vi "SO2 TCP Packet_v3.1.vi"(0 "ID":string, 5 "Version":string, 7 "TCP Packet In":string, 9 "utc_time":u32, 13 "Data Array":string[](array[string])) -> (8 "TCP Binary Packet":string)   [LabVIEW 2014]
panel:
  out "array":string[](array[string])
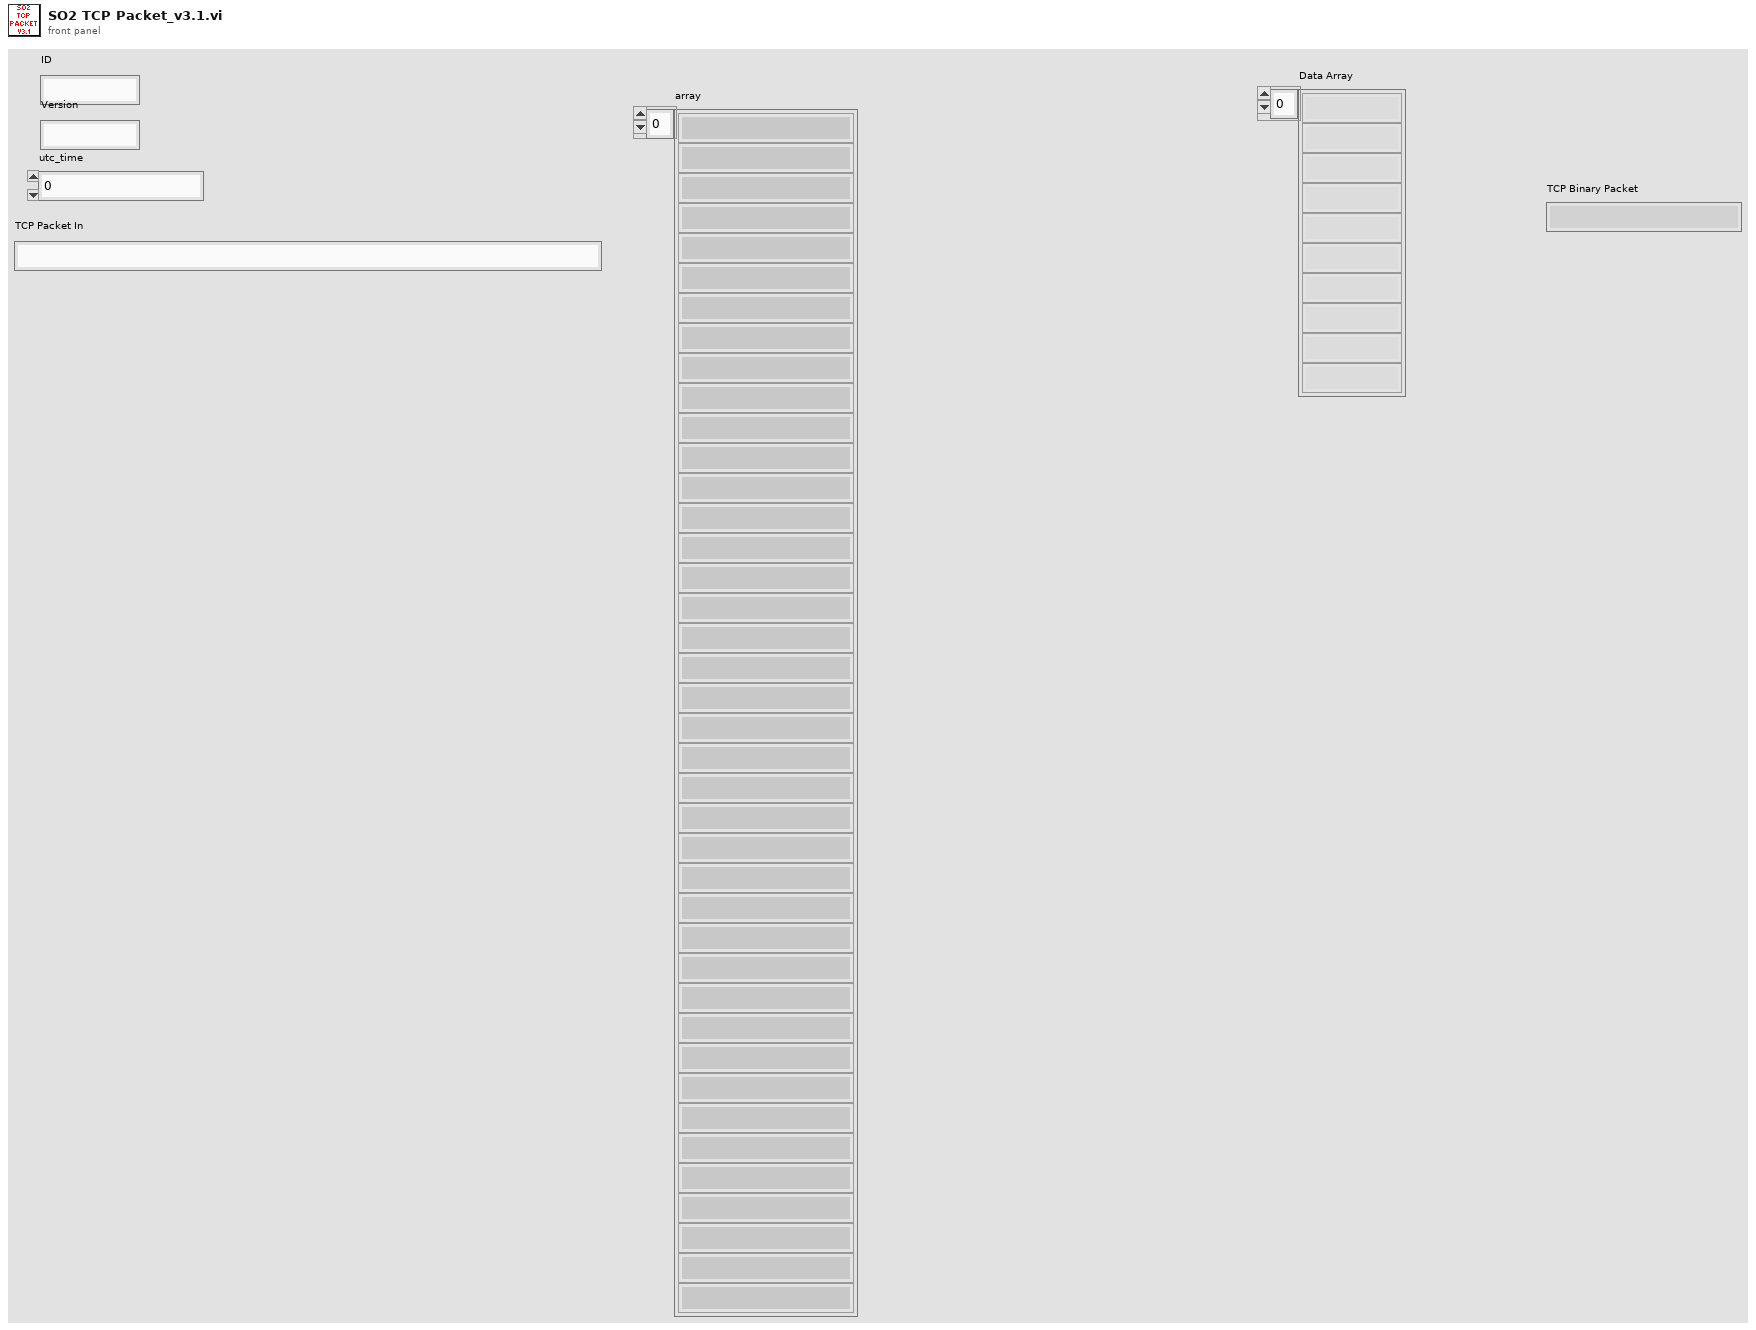
[diagram p1: front panel]
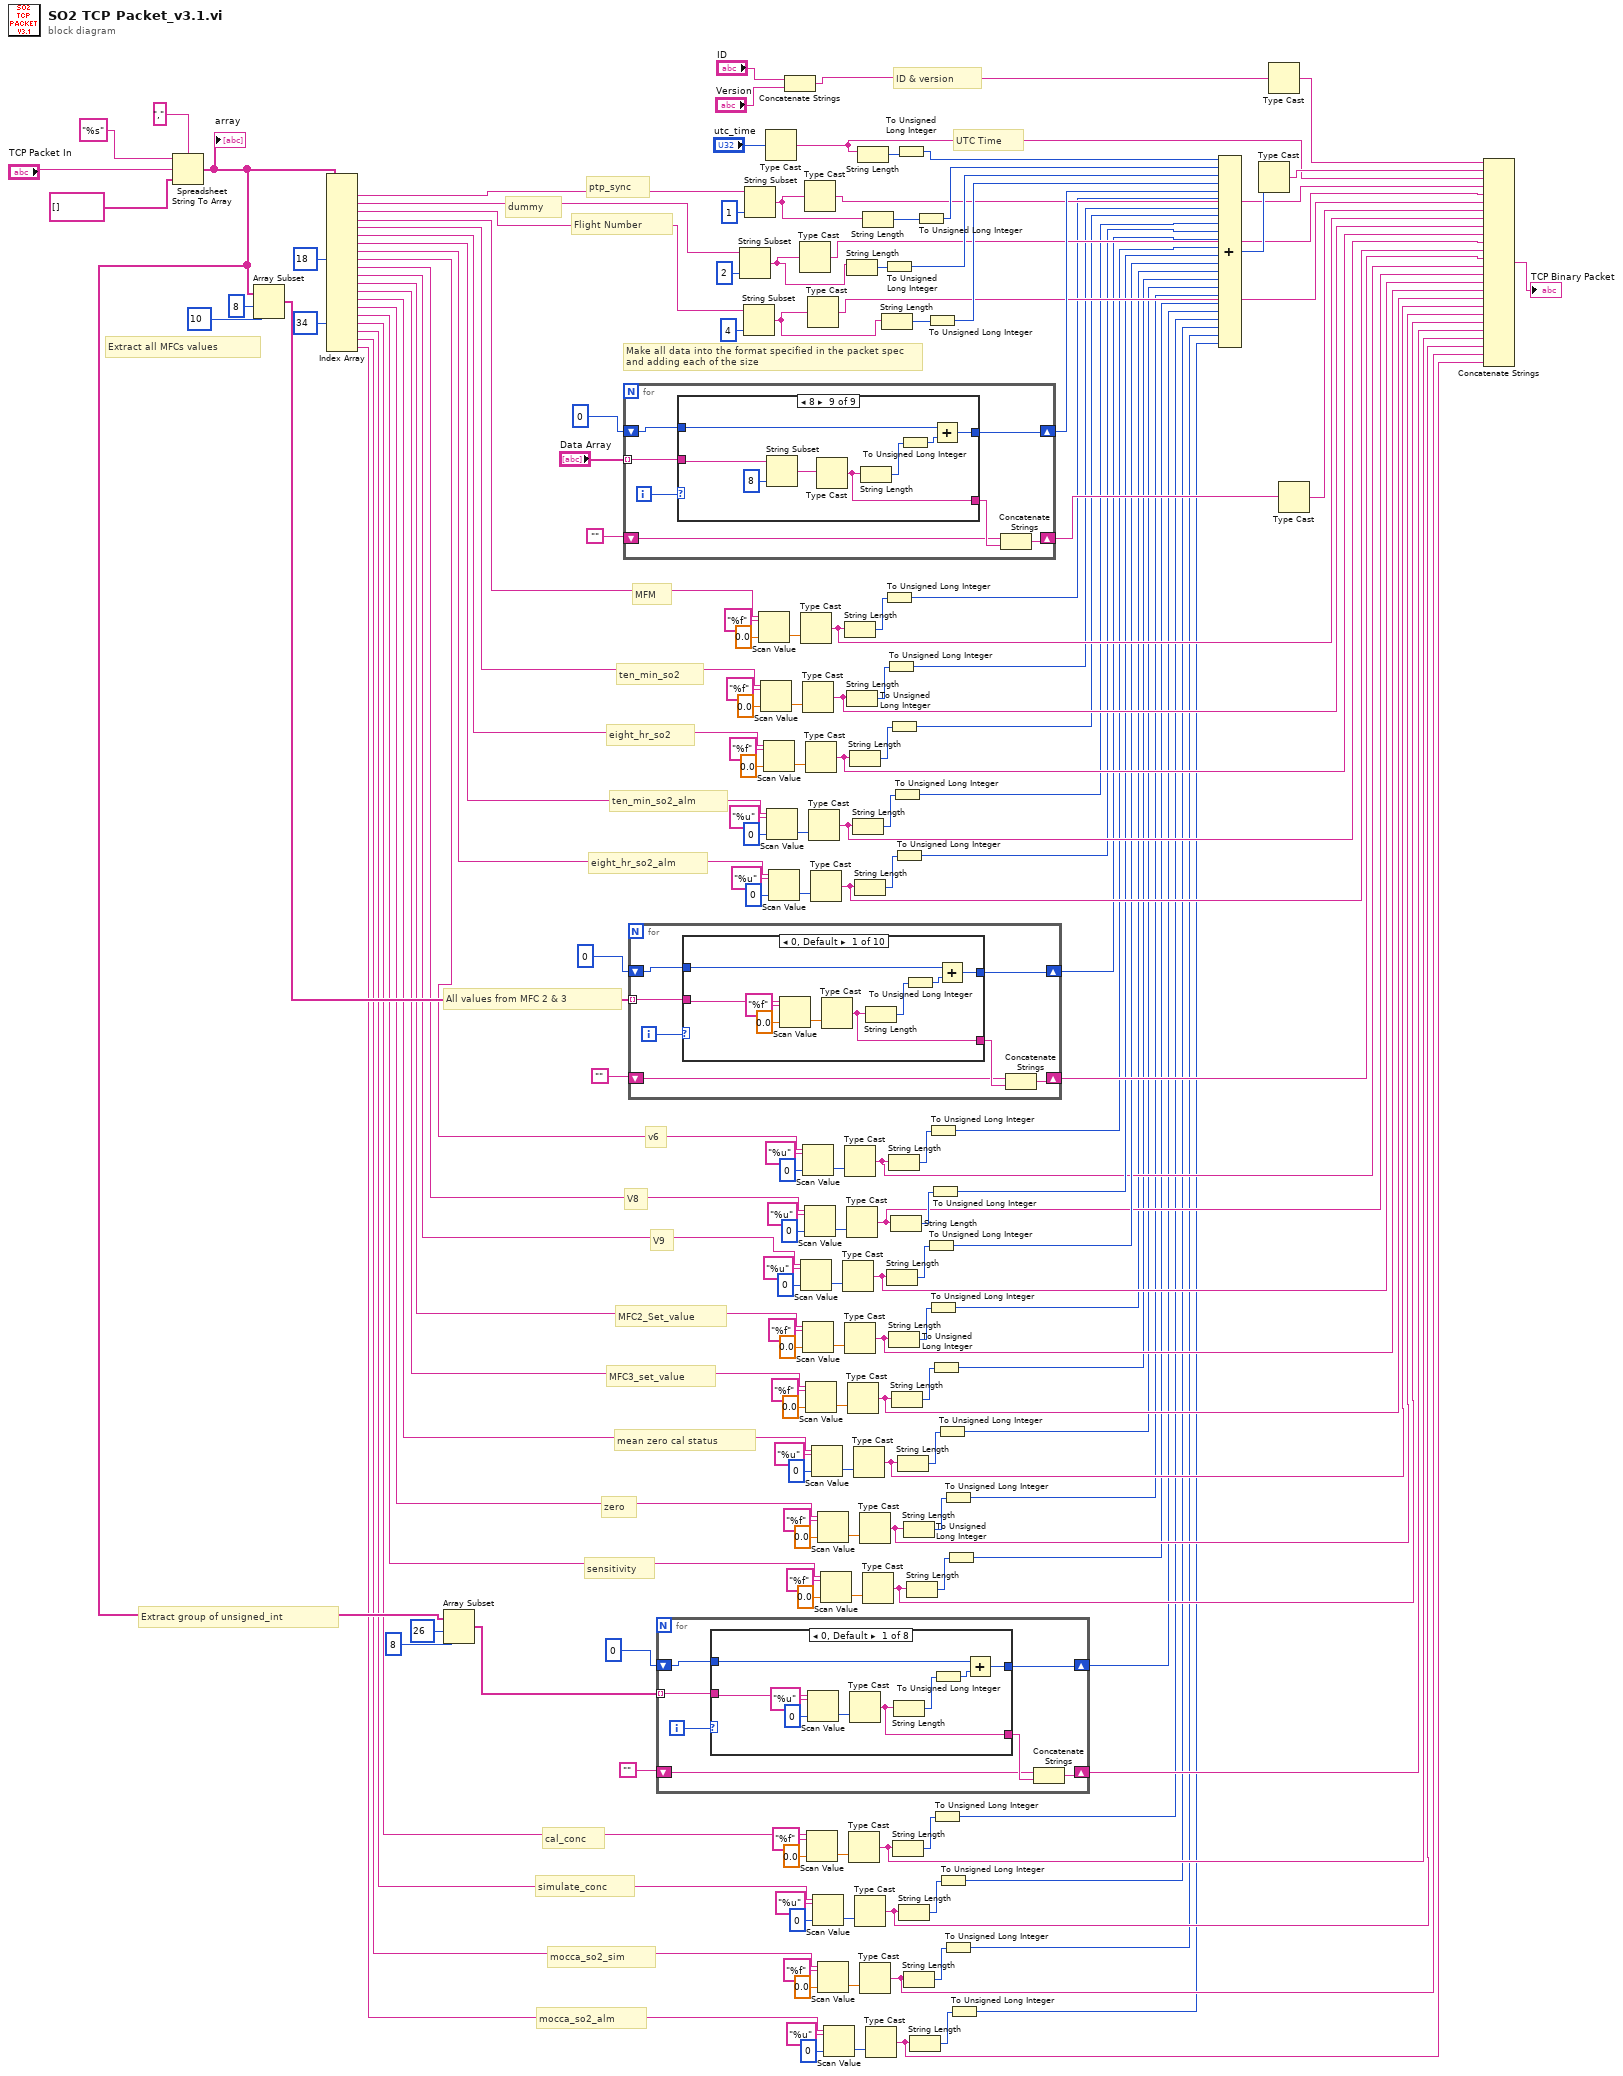
[diagram p0: block diagram]
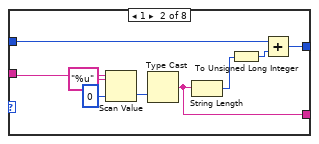
[diagram p2: hidden frame]
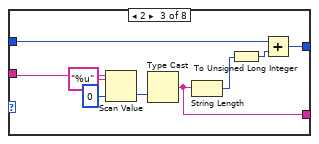
[diagram p3: hidden frame]
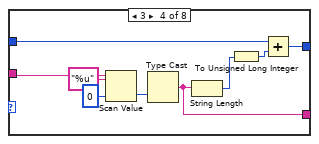
[diagram p4: hidden frame]
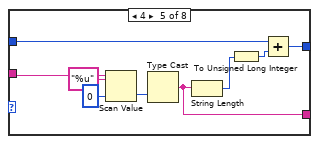
[diagram p5: hidden frame]
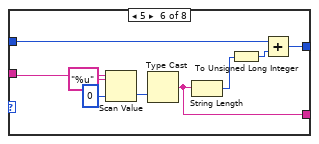
[diagram p6: hidden frame]
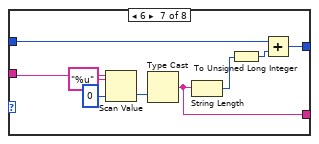
[diagram p7: hidden frame]
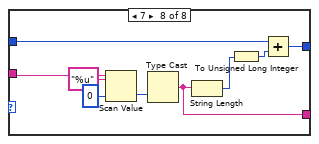
[diagram p8: hidden frame]
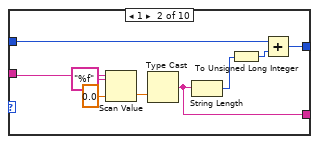
[diagram p9: hidden frame]
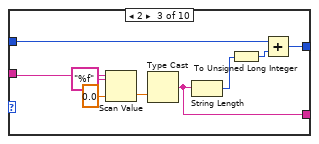
[diagram p10: hidden frame]
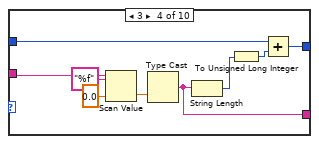
[diagram p11: hidden frame]
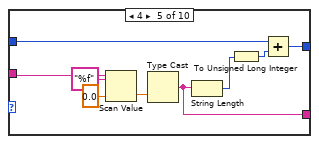
[diagram p12: hidden frame]
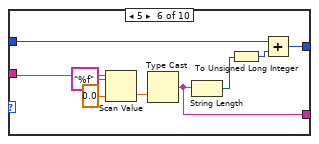
[diagram p13: hidden frame]
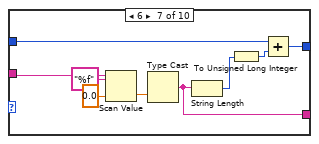
[diagram p14: hidden frame]
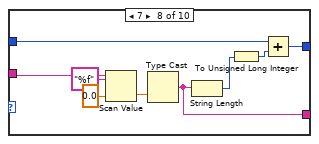
[diagram p15: hidden frame]
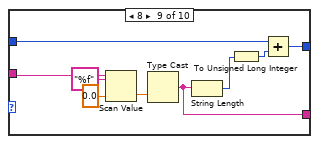
[diagram p16: hidden frame]
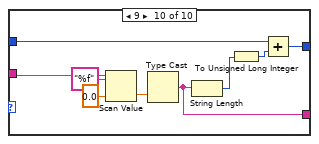
[diagram p17: hidden frame]
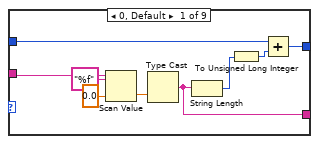
[diagram p18: hidden frame]
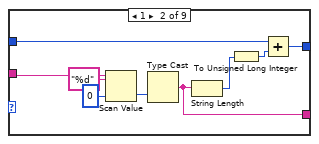
[diagram p19: hidden frame]
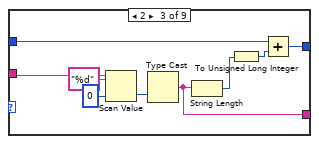
[diagram p20: hidden frame]
diagram:
  # "mocca_so2_alm"
  # "mocca_so2_sim"
  # "simulate_conc"
  # "cal_conc"
  # "Extract group of unsigned_int"
  # "sensitivity"
  # "zero"
  # "mean zero cal status"
  # "MFC3_set_value"
  # "MFC2_Set_value"
  # "V9"
  # "V8"
  # "v6"
  # "All values from MFC 2 & 3"
  # "Extract all MFCs values"
  # "eight_hr_so2_alm"
  # "ten_min_so2_alm"
  # "eight_hr_so2"
  # "ten_min_so2"
  # "MFM"
  # "Flight Number"
  # "dummy"
  # "ptp_sync"
  # "UTC Time"
  # "ID & version"
  # "Make all data into the format specified in the packet spec\nand adding each of the size"
  n1 = Spreadsheet String To Array(delimiter (Tab)=",", format string="%s", spreadsheet string="TCP Packet In", array type (2D Dbl)=string[] []) -> (array=w40:string[])
  "array" <- w40
  n2 = Array Subset(array=w40, index=8, length=10) -> (w102:string[])
  n3 = Index Array(array=w40, index #9=18 ("index"), index #17=34 ("index")) -> (element #1=w144:string, element #2=w143:string, element #3=w142:string, element #4=w137:string, element #5=w126:string, element #6=w123:string, element #7=w112:string, element #8=w109:string, element #9=w90:string, element #10=w89:string, element #11=w84:string, element #12=w69:string, element #13=w64:string, element #14=w59:string, element #15=w48:string, element #16=w43:string, element #17=w17:string, element #18=w8:string, element #19=w7:string, element #20=w6:string)  [unwired: 18 in]
  n4 = Array Subset(array=w40, index=26, length=8) -> (w36:string[])
  n5 = for {
    tunnel: "Data Array" -> [w181] mode=indexing
    shift-right: [w179] -> w163
    shift-left: u32 0 -> [w180]
    shift-right: [w178] -> w152
    shift-left: "" -> [w176]
    i -> [w182]
    n6 = case shown="8" w182 {
      tunnel: w181 -> [w189 w198 w207 w216 w225 w234 w243 w252 w256]
      tunnel: w180 -> [w187 w196 w205 w214 w223 w232 w241 w250 w262]
      tunnel: [w184 w193 w202 w211 w220 w229 w238 w247 w259] -> w179
      tunnel: [w183 w192 w201 w210 w219 w228 w237 w246 w258] -> w177
      frame 0, Default {
        n7 = Scan Value(string=w189, format string="%f", default (0 dbl)=sgl 0.0 ("default (0 I32)")) -> (value=w191:sgl)  [unwired: 1 out]
        n8 = Type Cast(x=w191) -> (*(type *) &x=w183:string)  [unwired: 1 in]
        n9 = String Length(string=w183) -> (length=w186:i32)
        n10 = To Unsigned Long Integer(number=w186) -> (unsigned 32bit integer=w185:u32)
        n11 = Add(x=w187, y=w185) -> (x+y=w184:u32)
      }
      frame 1 {
        n12 = Scan Value(string=w198, format string="%d", default (0 dbl)=0 ("default (0 I32)")) -> (value=w200:i32)  [unwired: 1 out]
        n13 = Type Cast(x=w200) -> (*(type *) &x=w192:string)  [unwired: 1 in]
        n14 = String Length(string=w192) -> (length=w195:i32)
        n15 = To Unsigned Long Integer(number=w195) -> (unsigned 32bit integer=w194:u32)
        n16 = Add(x=w196, y=w194) -> (x+y=w193:u32)
      }
      frame 2 {
        n17 = Scan Value(string=w207, format string="%d", default (0 dbl)=0 ("default (0 I32)")) -> (value=w209:i32)  [unwired: 1 out]
        n18 = Type Cast(x=w209) -> (*(type *) &x=w201:string)  [unwired: 1 in]
        n19 = String Length(string=w201) -> (length=w204:i32)
        n20 = To Unsigned Long Integer(number=w204) -> (unsigned 32bit integer=w203:u32)
        n21 = Add(x=w205, y=w203) -> (x+y=w202:u32)
      }
      frame 3 {
        n22 = Scan Value(string=w216, format string="%d", default (0 dbl)=0 ("default (0 I32)")) -> (value=w218:i32)  [unwired: 1 out]
        n23 = Type Cast(x=w218) -> (*(type *) &x=w210:string)  [unwired: 1 in]
        n24 = String Length(string=w210) -> (length=w213:i32)
        n25 = To Unsigned Long Integer(number=w213) -> (unsigned 32bit integer=w212:u32)
        n26 = Add(x=w214, y=w212) -> (x+y=w211:u32)
      }
      frame 4 {
        n27 = Scan Value(string=w225, format string="%f", default (0 dbl)=sgl 0.0 ("default (0 I32)")) -> (value=w227:sgl)  [unwired: 1 out]
        n28 = Type Cast(x=w227) -> (*(type *) &x=w219:string)  [unwired: 1 in]
        n29 = String Length(string=w219) -> (length=w222:i32)
        n30 = To Unsigned Long Integer(number=w222) -> (unsigned 32bit integer=w221:u32)
        n31 = Add(x=w223, y=w221) -> (x+y=w220:u32)
      }
      frame 5 {
        n32 = Scan Value(string=w234, format string="%f", default (0 dbl)=sgl 0.0 ("default (0 I32)")) -> (value=w236:sgl)  [unwired: 1 out]
        n33 = Type Cast(x=w236) -> (*(type *) &x=w228:string)  [unwired: 1 in]
        n34 = String Length(string=w228) -> (length=w231:i32)
        n35 = To Unsigned Long Integer(number=w231) -> (unsigned 32bit integer=w230:u32)
        n36 = Add(x=w232, y=w230) -> (x+y=w229:u32)
      }
      frame 6 {
        n37 = Scan Value(string=w243, format string="%f", default (0 dbl)=sgl 0.0 ("default (0 I32)")) -> (value=w245:sgl)  [unwired: 1 out]
        n38 = Type Cast(x=w245) -> (*(type *) &x=w237:string)  [unwired: 1 in]
        n39 = String Length(string=w237) -> (length=w240:i32)
        n40 = To Unsigned Long Integer(number=w240) -> (unsigned 32bit integer=w239:u32)
        n41 = Add(x=w241, y=w239) -> (x+y=w238:u32)
      }
      frame 7 {
        n42 = Scan Value(string=w252, format string="%f", default (0 dbl)=sgl 0.0 ("default (0 I32)")) -> (value=w254:sgl)  [unwired: 1 out]
        n43 = Type Cast(x=w254) -> (*(type *) &x=w246:string)  [unwired: 1 in]
        n44 = String Length(string=w246) -> (length=w249:i32)
        n45 = To Unsigned Long Integer(number=w249) -> (unsigned 32bit integer=w248:u32)
        n46 = Add(x=w250, y=w248) -> (x+y=w247:u32)
      }
      frame 8 {
        n47 = String Subset(string=w256, length (rest)=8 ("length (rest)")) -> (substring=w255:string)  [unwired: 1 in]
        n48 = Type Cast(x=w255) -> (*(type *) &x=w258:string)  [unwired: 1 in]
        n49 = String Length(string=w258) -> (length=w261:i32)
        n50 = To Unsigned Long Integer(number=w261) -> (unsigned 32bit integer=w260:u32)
        n51 = Add(x=w262, y=w260) -> (x+y=w259:u32)
      }
    }
    n52 = Concatenate Strings(w176, w177) -> (w178:string)
  }
  n53 = for {
    tunnel: w102 -> [w268] mode=indexing
    shift-right: [w266] -> w101
    shift-left: u32 0 -> [w267]
    shift-right: [w265] -> w100
    shift-left: "" -> [w263]
    i -> [w269]
    n54 = case shown="0, Default" w269 {
      tunnel: w268 -> [w276 w285 w294 w303 w312 w321 w330 w339 w348 w357]
      tunnel: w267 -> [w274 w283 w292 w301 w310 w319 w328 w337 w346 w355]
      tunnel: [w271 w280 w289 w298 w307 w316 w325 w334 w343 w352] -> w266
      tunnel: [w270 w279 w288 w297 w306 w315 w324 w333 w342 w351] -> w264
      frame 0, Default {
        n55 = Scan Value(string=w276, format string="%f", default (0 dbl)=sgl 0.0 ("default (0 I32)")) -> (value=w278:sgl)  [unwired: 1 out]
        n56 = Type Cast(x=w278) -> (*(type *) &x=w270:string)  [unwired: 1 in]
        n57 = String Length(string=w270) -> (length=w273:i32)
        n58 = To Unsigned Long Integer(number=w273) -> (unsigned 32bit integer=w272:u32)
        n59 = Add(x=w274, y=w272) -> (x+y=w271:u32)
      }
      frame 1 {
        n60 = Scan Value(string=w285, format string="%f", default (0 dbl)=sgl 0.0 ("default (0 I32)")) -> (value=w287:sgl)  [unwired: 1 out]
        n61 = Type Cast(x=w287) -> (*(type *) &x=w279:string)  [unwired: 1 in]
        n62 = String Length(string=w279) -> (length=w282:i32)
        n63 = To Unsigned Long Integer(number=w282) -> (unsigned 32bit integer=w281:u32)
        n64 = Add(x=w283, y=w281) -> (x+y=w280:u32)
      }
      frame 2 {
        n65 = Scan Value(string=w294, format string="%f", default (0 dbl)=sgl 0.0 ("default (0 I32)")) -> (value=w296:sgl)  [unwired: 1 out]
        n66 = Type Cast(x=w296) -> (*(type *) &x=w288:string)  [unwired: 1 in]
        n67 = String Length(string=w288) -> (length=w291:i32)
        n68 = To Unsigned Long Integer(number=w291) -> (unsigned 32bit integer=w290:u32)
        n69 = Add(x=w292, y=w290) -> (x+y=w289:u32)
      }
      frame 3 {
        n70 = Scan Value(string=w303, format string="%f", default (0 dbl)=sgl 0.0 ("default (0 I32)")) -> (value=w305:sgl)  [unwired: 1 out]
        n71 = Type Cast(x=w305) -> (*(type *) &x=w297:string)  [unwired: 1 in]
        n72 = String Length(string=w297) -> (length=w300:i32)
        n73 = To Unsigned Long Integer(number=w300) -> (unsigned 32bit integer=w299:u32)
        n74 = Add(x=w301, y=w299) -> (x+y=w298:u32)
      }
      frame 4 {
        n75 = Scan Value(string=w312, format string="%f", default (0 dbl)=sgl 0.0 ("default (0 I32)")) -> (value=w314:sgl)  [unwired: 1 out]
        n76 = Type Cast(x=w314) -> (*(type *) &x=w306:string)  [unwired: 1 in]
        n77 = String Length(string=w306) -> (length=w309:i32)
        n78 = To Unsigned Long Integer(number=w309) -> (unsigned 32bit integer=w308:u32)
        n79 = Add(x=w310, y=w308) -> (x+y=w307:u32)
      }
      frame 5 {
        n80 = Scan Value(string=w321, format string="%f", default (0 dbl)=sgl 0.0 ("default (0 I32)")) -> (value=w323:sgl)  [unwired: 1 out]
        n81 = Type Cast(x=w323) -> (*(type *) &x=w315:string)  [unwired: 1 in]
        n82 = String Length(string=w315) -> (length=w318:i32)
        n83 = To Unsigned Long Integer(number=w318) -> (unsigned 32bit integer=w317:u32)
        n84 = Add(x=w319, y=w317) -> (x+y=w316:u32)
      }
      frame 6 {
        n85 = Scan Value(string=w330, format string="%f", default (0 dbl)=sgl 0.0 ("default (0 I32)")) -> (value=w332:sgl)  [unwired: 1 out]
        n86 = Type Cast(x=w332) -> (*(type *) &x=w324:string)  [unwired: 1 in]
        n87 = String Length(string=w324) -> (length=w327:i32)
        n88 = To Unsigned Long Integer(number=w327) -> (unsigned 32bit integer=w326:u32)
        n89 = Add(x=w328, y=w326) -> (x+y=w325:u32)
      }
      frame 7 {
        n90 = Scan Value(string=w339, format string="%f", default (0 dbl)=sgl 0.0 ("default (0 I32)")) -> (value=w341:sgl)  [unwired: 1 out]
        n91 = Type Cast(x=w341) -> (*(type *) &x=w333:string)  [unwired: 1 in]
        n92 = String Length(string=w333) -> (length=w336:i32)
        n93 = To Unsigned Long Integer(number=w336) -> (unsigned 32bit integer=w335:u32)
        n94 = Add(x=w337, y=w335) -> (x+y=w334:u32)
      }
      frame 8 {
        n95 = Scan Value(string=w348, format string="%f", default (0 dbl)=sgl 0.0 ("default (0 I32)")) -> (value=w350:sgl)  [unwired: 1 out]
        n96 = Type Cast(x=w350) -> (*(type *) &x=w342:string)  [unwired: 1 in]
        n97 = String Length(string=w342) -> (length=w345:i32)
        n98 = To Unsigned Long Integer(number=w345) -> (unsigned 32bit integer=w344:u32)
        n99 = Add(x=w346, y=w344) -> (x+y=w343:u32)
      }
      frame 9 {
        n100 = Scan Value(string=w357, format string="%f", default (0 dbl)=sgl 0.0 ("default (0 I32)")) -> (value=w359:sgl)  [unwired: 1 out]
        n101 = Type Cast(x=w359) -> (*(type *) &x=w351:string)  [unwired: 1 in]
        n102 = String Length(string=w351) -> (length=w354:i32)
        n103 = To Unsigned Long Integer(number=w354) -> (unsigned 32bit integer=w353:u32)
        n104 = Add(x=w355, y=w353) -> (x+y=w352:u32)
      }
    }
    n105 = Concatenate Strings(w263, w264) -> (w265:string)
  }
  n106 = for {
    tunnel: w36 -> [w365] mode=indexing
    shift-right: [w363] -> w35
    shift-left: u32 0 -> [w364]
    shift-right: [w362] -> w34
    shift-left: "" -> [w360]
    i -> [w366]
    n107 = case shown="0, Default" w366 {
      tunnel: w365 -> [w373 w382 w391 w400 w409 w418 w427 w436]
      tunnel: w364 -> [w371 w380 w389 w398 w407 w416 w425 w434]
      tunnel: [w368 w377 w386 w395 w404 w413 w422 w431] -> w363
      tunnel: [w367 w376 w385 w394 w403 w412 w421 w430] -> w361
      frame 0, Default {
        n108 = Scan Value(string=w373, format string="%u", default (0 dbl)=u16 0 ("default (0 I32)")) -> (value=w375:u16)  [unwired: 1 out]
        n109 = Type Cast(x=w375) -> (*(type *) &x=w367:string)  [unwired: 1 in]
        n110 = String Length(string=w367) -> (length=w370:i32)
        n111 = To Unsigned Long Integer(number=w370) -> (unsigned 32bit integer=w369:u32)
        n112 = Add(x=w371, y=w369) -> (x+y=w368:u32)
      }
      frame 1 {
        n113 = Scan Value(string=w382, format string="%u", default (0 dbl)=u16 0 ("default (0 I32)")) -> (value=w384:u16)  [unwired: 1 out]
        n114 = Type Cast(x=w384) -> (*(type *) &x=w376:string)  [unwired: 1 in]
        n115 = String Length(string=w376) -> (length=w379:i32)
        n116 = To Unsigned Long Integer(number=w379) -> (unsigned 32bit integer=w378:u32)
        n117 = Add(x=w380, y=w378) -> (x+y=w377:u32)
      }
      frame 2 {
        n118 = Scan Value(string=w391, format string="%u", default (0 dbl)=u16 0 ("default (0 I32)")) -> (value=w393:u16)  [unwired: 1 out]
        n119 = Type Cast(x=w393) -> (*(type *) &x=w385:string)  [unwired: 1 in]
        n120 = String Length(string=w385) -> (length=w388:i32)
        n121 = To Unsigned Long Integer(number=w388) -> (unsigned 32bit integer=w387:u32)
        n122 = Add(x=w389, y=w387) -> (x+y=w386:u32)
      }
      frame 3 {
        n123 = Scan Value(string=w400, format string="%u", default (0 dbl)=u16 0 ("default (0 I32)")) -> (value=w402:u16)  [unwired: 1 out]
        n124 = Type Cast(x=w402) -> (*(type *) &x=w394:string)  [unwired: 1 in]
        n125 = String Length(string=w394) -> (length=w397:i32)
        n126 = To Unsigned Long Integer(number=w397) -> (unsigned 32bit integer=w396:u32)
        n127 = Add(x=w398, y=w396) -> (x+y=w395:u32)
      }
      frame 4 {
        n128 = Scan Value(string=w409, format string="%u", default (0 dbl)=u16 0 ("default (0 I32)")) -> (value=w411:u16)  [unwired: 1 out]
        n129 = Type Cast(x=w411) -> (*(type *) &x=w403:string)  [unwired: 1 in]
        n130 = String Length(string=w403) -> (length=w406:i32)
        n131 = To Unsigned Long Integer(number=w406) -> (unsigned 32bit integer=w405:u32)
        n132 = Add(x=w407, y=w405) -> (x+y=w404:u32)
      }
      frame 5 {
        n133 = Scan Value(string=w418, format string="%u", default (0 dbl)=u16 0 ("default (0 I32)")) -> (value=w420:u16)  [unwired: 1 out]
        n134 = Type Cast(x=w420) -> (*(type *) &x=w412:string)  [unwired: 1 in]
        n135 = String Length(string=w412) -> (length=w415:i32)
        n136 = To Unsigned Long Integer(number=w415) -> (unsigned 32bit integer=w414:u32)
        n137 = Add(x=w416, y=w414) -> (x+y=w413:u32)
      }
      frame 6 {
        n138 = Scan Value(string=w427, format string="%u", default (0 dbl)=u16 0 ("default (0 I32)")) -> (value=w429:u16)  [unwired: 1 out]
        n139 = Type Cast(x=w429) -> (*(type *) &x=w421:string)  [unwired: 1 in]
        n140 = String Length(string=w421) -> (length=w424:i32)
        n141 = To Unsigned Long Integer(number=w424) -> (unsigned 32bit integer=w423:u32)
        n142 = Add(x=w425, y=w423) -> (x+y=w422:u32)
      }
      frame 7 {
        n143 = Scan Value(string=w436, format string="%u", default (0 dbl)=u16 0 ("default (0 I32)")) -> (value=w438:u16)  [unwired: 1 out]
        n144 = Type Cast(x=w438) -> (*(type *) &x=w430:string)  [unwired: 1 in]
        n145 = String Length(string=w430) -> (length=w433:i32)
        n146 = To Unsigned Long Integer(number=w433) -> (unsigned 32bit integer=w432:u32)
        n147 = Add(x=w434, y=w432) -> (x+y=w431:u32)
      }
    }
    n148 = Concatenate Strings(w360, w361) -> (w362:string)
  }
  n149 = String Subset(string=w143, length (rest)=2 ("length (rest)")) -> (substring=w150:string)  [unwired: 1 in]
  n150 = String Subset(string=w142, length (rest)=4 ("length (rest)")) -> (substring=w156:string)  [unwired: 1 in]
  n151 = String Subset(string=w144, length (rest)=1 ("length (rest)")) -> (substring=w159:string)  [unwired: 1 in]
  n152 = Scan Value(string=w137, format string="%f", default (0 dbl)=sgl 0.0 ("default (0 I32)")) -> (value=w141:sgl)  [unwired: 1 out]
  n153 = Scan Value(string=w126, format string="%f", default (0 dbl)=sgl 0.0 ("default (0 I32)")) -> (value=w134:sgl)  [unwired: 1 out]
  n154 = Scan Value(string=w123, format string="%f", default (0 dbl)=sgl 0.0 ("default (0 I32)")) -> (value=w130:sgl)  [unwired: 1 out]
  n155 = Type Cast(x="utc_time") -> (*(type *) &x=w1:string)  [unwired: 1 in]
  n156 = Scan Value(string=w112, format string="%u", default (0 dbl)=u16 0 ("default (0 I32)")) -> (value=w120:u16)  [unwired: 1 out]
  n157 = Scan Value(string=w109, format string="%u", default (0 dbl)=u16 0 ("default (0 I32)")) -> (value=w116:u16)  [unwired: 1 out]
  n158 = Concatenate Strings("ID", "Version") -> (w2:string)
  n159 = Type Cast(x=w150) -> (*(type *) &x=w149:string)  [unwired: 1 in]
  n160 = Type Cast(x=w141) -> (*(type *) &x=w135:string)  [unwired: 1 in]
  n161 = Scan Value(string=w84, format string="%u", default (0 dbl)=u16 0 ("default (0 I32)")) -> (value=w88:u16)  [unwired: 1 out]
  n162 = Type Cast(x=w134) -> (*(type *) &x=w124:string)  [unwired: 1 in]
  n163 = Scan Value(string=w90, format string="%u", default (0 dbl)=u16 0 ("default (0 I32)")) -> (value=w98:u16)  [unwired: 1 out]
  n164 = Scan Value(string=w69, format string="%f", default (0 dbl)=sgl 0.0 ("default (0 I32)")) -> (value=w77:sgl)  [unwired: 1 out]
  n165 = Type Cast(x=w159) -> (*(type *) &x=w158:string)  [unwired: 1 in]
  n166 = Scan Value(string=w89, format string="%u", default (0 dbl)=u16 0 ("default (0 I32)")) -> (value=w94:u16)  [unwired: 1 out]
  n167 = Type Cast(x=w130) -> (*(type *) &x=w121:string)  [unwired: 1 in]
  n168 = Scan Value(string=w64, format string="%f", default (0 dbl)=sgl 0.0 ("default (0 I32)")) -> (value=w73:sgl)  [unwired: 1 out]
  n169 = Scan Value(string=w17, format string="%f", default (0 dbl)=sgl 0.0 ("default (0 I32)")) -> (value=w33:sgl)  [unwired: 1 out]
  n170 = Type Cast(x=w156) -> (*(type *) &x=w157:string)  [unwired: 1 in]
  n171 = Type Cast(x=w120) -> (*(type *) &x=w110:string)  [unwired: 1 in]
  n172 = Type Cast(x=w116) -> (*(type *) &x=w107:string)  [unwired: 1 in]
  n173 = Scan Value(string=w59, format string="%u", default (0 dbl)=u16 0 ("default (0 I32)")) -> (value=w63:u16)  [unwired: 1 out]
  n174 = Scan Value(string=w8, format string="%u", default (0 dbl)=u16 0 ("default (0 I32)")) -> (value=w29:u16)  [unwired: 1 out]
  n175 = Scan Value(string=w48, format string="%f", default (0 dbl)=sgl 0.0 ("default (0 I32)")) -> (value=w56:sgl)  [unwired: 1 out]
  n176 = Scan Value(string=w7, format string="%f", default (0 dbl)=sgl 0.0 ("default (0 I32)")) -> (value=w25:sgl)  [unwired: 1 out]
  n177 = Scan Value(string=w43, format string="%f", default (0 dbl)=sgl 0.0 ("default (0 I32)")) -> (value=w52:sgl)  [unwired: 1 out]
  n178 = Scan Value(string=w6, format string="%u", default (0 dbl)=u16 0 ("default (0 I32)")) -> (value=w21:u16)  [unwired: 1 out]
  n179 = Type Cast(x=w88) -> (*(type *) &x=w78:string)  [unwired: 1 in]
  n180 = String Length(string=w135) -> (length=w138:i32)
  n181 = Type Cast(x=w98) -> (*(type *) &x=w80:string)  [unwired: 1 in]
  n182 = Type Cast(x=w77) -> (*(type *) &x=w67:string)  [unwired: 1 in]
  n183 = String Length(string=w150) -> (length=w170:i32)
  n184 = String Length(string=w124) -> (length=w131:i32)
  n185 = Type Cast(x=w94) -> (*(type *) &x=w79:string)  [unwired: 1 in]
  n186 = Type Cast(x=w73) -> (*(type *) &x=w65:string)  [unwired: 1 in]
  n187 = Type Cast(x=w33) -> (*(type *) &x=w15:string)  [unwired: 1 in]
  n188 = String Length(string=w121) -> (length=w127:i32)
  n189 = String Length(string=w110) -> (length=w117:i32)
  n190 = Type Cast(x=w63) -> (*(type *) &x=w57:string)  [unwired: 1 in]
  n191 = String Length(string=w107) -> (length=w113:i32)
  n192 = Type Cast(x=w29) -> (*(type *) &x=w13:string)  [unwired: 1 in]
  n193 = String Length(string=w1) -> (length=w175:i32)
  n194 = Type Cast(x=w56) -> (*(type *) &x=w46:string)  [unwired: 1 in]
  n195 = Type Cast(x=w25) -> (*(type *) &x=w11:string)  [unwired: 1 in]
  n196 = String Length(string=w159) -> (length=w172:i32)
  n197 = Type Cast(x=w52) -> (*(type *) &x=w44:string)  [unwired: 1 in]
  n198 = Type Cast(x=w21) -> (*(type *) &x=w9:string)  [unwired: 1 in]
  n199 = String Length(string=w156) -> (length=w167:i32)
  n200 = To Unsigned Long Integer(number=w170) -> (unsigned 32bit integer=w169:u32)
  n201 = To Unsigned Long Integer(number=w138) -> (unsigned 32bit integer=w136:u32)
  n202 = To Unsigned Long Integer(number=w131) -> (unsigned 32bit integer=w125:u32)
  n203 = String Length(string=w78) -> (length=w85:i32)
  n204 = To Unsigned Long Integer(number=w127) -> (unsigned 32bit integer=w122:u32)
  n205 = String Length(string=w80) -> (length=w95:i32)
  n206 = String Length(string=w67) -> (length=w74:i32)
  n207 = String Length(string=w79) -> (length=w91:i32)
  n208 = To Unsigned Long Integer(number=w117) -> (unsigned 32bit integer=w111:u32)
  n209 = String Length(string=w65) -> (length=w70:i32)
  n210 = String Length(string=w15) -> (length=w30:i32)
  n211 = To Unsigned Long Integer(number=w113) -> (unsigned 32bit integer=w108:u32)
  n212 = To Unsigned Long Integer(number=w175) -> (unsigned 32bit integer=w174:u32)
  n213 = String Length(string=w57) -> (length=w60:i32)
  n214 = String Length(string=w13) -> (length=w26:i32)
  n215 = String Length(string=w46) -> (length=w53:i32)
  n216 = String Length(string=w11) -> (length=w22:i32)
  n217 = String Length(string=w44) -> (length=w49:i32)
  n218 = String Length(string=w9) -> (length=w18:i32)
  n219 = To Unsigned Long Integer(number=w172) -> (unsigned 32bit integer=w171:u32)
  n220 = To Unsigned Long Integer(number=w85) -> (unsigned 32bit integer=w81:u32)
  n221 = To Unsigned Long Integer(number=w167) -> (unsigned 32bit integer=w166:u32)
  n222 = To Unsigned Long Integer(number=w95) -> (unsigned 32bit integer=w83:u32)
  n223 = To Unsigned Long Integer(number=w74) -> (unsigned 32bit integer=w68:u32)
  n224 = To Unsigned Long Integer(number=w91) -> (unsigned 32bit integer=w82:u32)
  n225 = To Unsigned Long Integer(number=w70) -> (unsigned 32bit integer=w66:u32)
  n226 = To Unsigned Long Integer(number=w30) -> (unsigned 32bit integer=w16:u32)
  n227 = To Unsigned Long Integer(number=w60) -> (unsigned 32bit integer=w58:u32)
  n228 = To Unsigned Long Integer(number=w26) -> (unsigned 32bit integer=w14:u32)
  n229 = To Unsigned Long Integer(number=w53) -> (unsigned 32bit integer=w47:u32)
  n230 = To Unsigned Long Integer(number=w22) -> (unsigned 32bit integer=w12:u32)
  n231 = To Unsigned Long Integer(number=w49) -> (unsigned 32bit integer=w45:u32)
  n232 = To Unsigned Long Integer(number=w18) -> (unsigned 32bit integer=w10:u32)
  n233 = Compound Arithmetic op=ADD(w174, w171, w169, w166, w163, w136, w125, w122, w111, w108, w101, w83, w82, w81, w68, w66, w58, w47, w45, w35, w16, w14, w12, w10) -> (w161:u32)
  n234 = Type Cast(x=w161) -> (*(type *) &x=w160:string)  [unwired: 1 in]
  n235 = Type Cast(x=w2) -> (*(type *) &x=w162:string)  [unwired: 1 in]
  n236 = Type Cast(x=w152) -> (*(type *) &x=w155:string)  [unwired: 1 in]
  n237 = Concatenate Strings(w162, w160, w1, w158, w149, w157, w155, w135, w124, w121, w110, w107, w100, w80, w79, w78, w67, w65, w57, w46, w44, w34, w15, w13, w11, w9) -> (→"TCP Binary Packet":string)
